vi "单槽配方预览.vi"(11 "数组":variant[](array[variant])) -> (3 "返回数据":variant[](array[variant]))   [LabVIEW 2013]
panel:
  in  "返回编辑":bool
  in  "确认配方":bool
  in  "配方预览":string[][](table)=[["工序01", "前轴定位器", "", "", "", "", "", "", "", "", ""], ["工序02", "前处理", "", "", "", "", "", "", "", "", ""], ["", "虹吸时间", "总时间", "", "", "", "", "", "", "", ""], ["第一步", "", "11", "", "", "", "", "", "", "", ""], ["工序03", "镀铜槽", "", "", "", "", "", "", "", "", ""], ["", "电源1电流", "电源2电流", "添加剂流量", "旋转电机转速", "药液流量", "总时间", "", "", "", ""], ["第一步", "", "4", "5", "3", "2", "8", "", "", "", ""], ["工序04", "水洗槽", "", "", "", "", "", "", "", "", ""], ["", "左电机转速\n", "中电机转速\n", "右电机转速", "M/S供应运行时间\n", "DI供应运行时间\n", "回喷水运行时间\n", "HF供应运行时间", "SCI供应运行时间\n", "氮气运行时间\n", "总时间"], ["第一步", "7", "8", "9", "0.000000", "0.000000", "0.000000", "0.000000", "0.000000", "0.000000", "20"]]
  # "配方浏览"
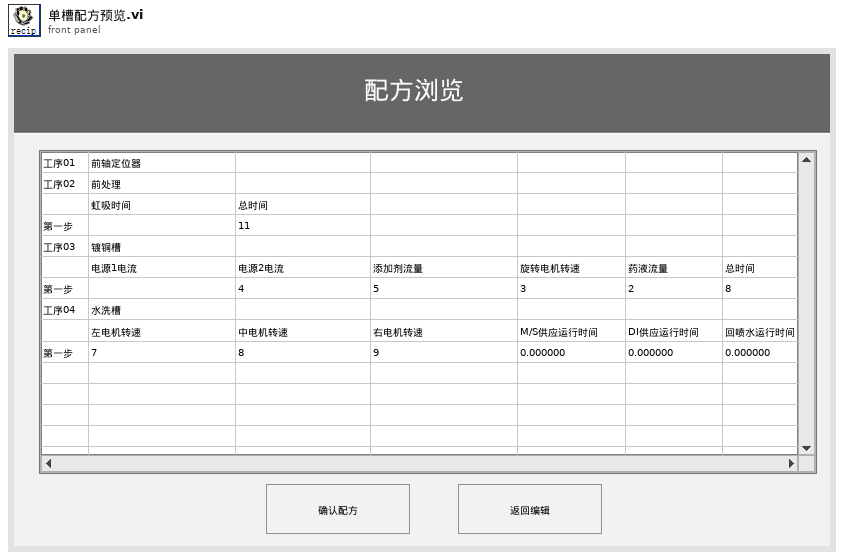
[diagram p1: front panel]
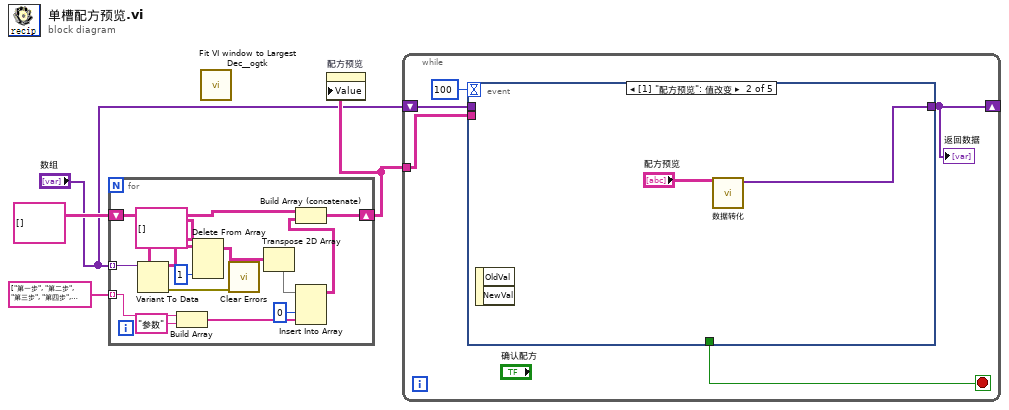
[diagram p0: block diagram]
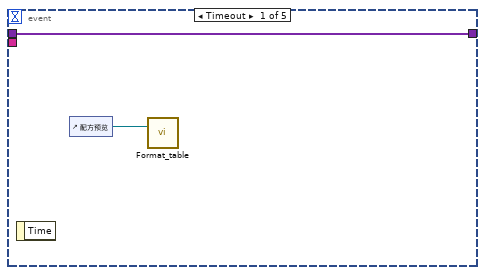
[diagram p2: hidden frame]
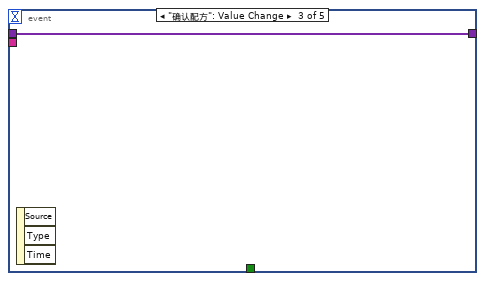
[diagram p3: hidden frame]
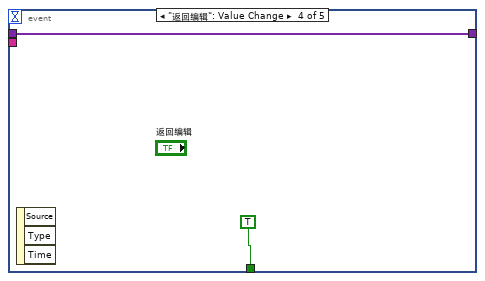
[diagram p4: hidden frame]
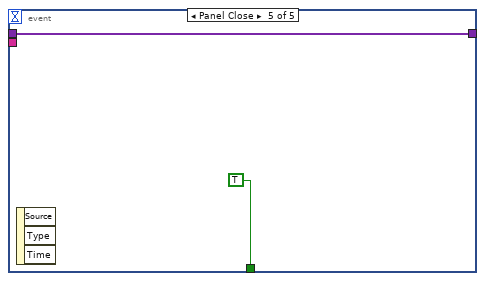
[diagram p5: hidden frame]
diagram:
  n1 = for {
    tunnel: "数组" -> [w16] mode=indexing
    shift-right: [w14] -> w2
    shift-left: string[][] [] -> [w15]
    tunnel: string[] ["第一步", "第二步", "第三步", "第四步", "第五步", "第六步", "第八步", "第九步", "第十步", "第十一步", "第十二步", "第十三步", "第十四步", "第十五步", "第十六步"] -> [w13] mode=indexing
    n2 = Variant To Data(type=string[][] [] ("已删除元素的数组子集"), Variant=w16) -> (data=w7:string[][], error out=w18:errorcluster)  [unwired: 1 in]
    n3 = Build Array(w13, "参数" ("元素")) -> (w10:string[])
    n4 = Delete From Array(array=w7, index (col)=1 ("禁用的索引 (列)")) -> (array with subset deleted=w6:string[][])  [unwired: 2 in, 1 out]
    n5 = call <vilib>:"Clear Errors.vi"("error in (no error)"=w18) -> ()  [unwired: 6 in, 1 out]
    n6 = Transpose 2D Array(2D array=w6) -> (transposed array=w11:string[][])
    n7 = Insert Into Array(array=w11, index (col)=0 ("禁用的索引 (列)"), new element=w10) -> (w8:string[][])  [unwired: 1 in]
    n8 = Build Array (concatenate)(w15, w8) -> (w14:string[][])
  }
  n9 = call <userlib>:"Fit VI window to Largest Dec__ogtk.vi"() -> ()  [unwired: 6 in, 2 out]
  n10 = property on="配方预览" class="Tbl (严格)"("Value"=w2) -> ()  [unwired: 2 in, 2 out]
  n11 = while {
    tunnel: w2 -> [w23]
    shift-right: [w21] -> _
    shift-left: "数组" -> [w22]
    stop <- w19 stop-if-true
    n12 = event shown="[1] \"配方预览\": 值改变" {
      selector: _ -> [_ _ _ _ _]
      dyn-events: _ -> [_ _ _ _ _]
      timeout: 100 -> [_ _ _ _ _]
      tunnel: w23 -> [_ _ _ _ _]
      tunnel: [_ _ _ TRUE TRUE] -> w19
      tunnel: w22 -> [w25 _ w28 w29 w31]
      tunnel: [w25 w26 w28 w29 w31] -> w21
      event Timeout {
        n13 = event-data() -> ()  [unwired: 1 in, 1 out]
        n14 = control-ref of="配方预览"() -> (w24:refnum<vi>)
        n15 = call "Format_table.vi"("Table Control"=w24) -> ()  [unwired: 2 in]
      }
      event "配方预览": Value Change {
        n16 = event-data() -> ()  [unwired: 1 in, 2 out]
        n17 = call "数据转化.vi"("配方数据"="配方预览") -> ("转化数据"=w26:variant[])  [unwired: 10 in]
      }
      event "确认配方": Value Change {
        n18 = event-data() -> ()  [unwired: 1 in, 3 out]
      }
      event "返回编辑": Value Change {
        n19 = event-data() -> ()  [unwired: 1 in, 3 out]
      }
      event Panel Close {
        n20 = event-data() -> ()  [unwired: 1 in, 3 out]
      }
    }
    "返回数据" <- w21
  }
